vi "Finish.vi"   [LabVIEW 2017]
doc: "This VI is called just before exiting. It is expected to close I/O refnum, save collected data, etc."
uses:
  <vilib>/Rock Robotics/WPI/Utilities/WPI_GetSetVariantRefNum.vi
types:
  T1 = typedef "WPI_MotorControlDeviceRef.ctl" = cluster{"DeviceStatus":errorcluster, "Type":T2, "PWM":cluster{"PWM Channel":T3, "DeadBand":T4}, "CAN":cluster{"Device Number":u8, "SetOutput VI Ref":variant, "GetOutput VI Ref":variant, "Enable VI Ref":variant, "Disable VI Ref":variant, "Data":variant}, "Invert":bool, "DIO PWM":cluster{"PWM \"Enable\" Channel":T3, "DIOChannel":T5, "PWM Rate":dbl}}
  T2 = typedef "WPI_MotorControlType.ctl" = enum16{"PWM", "CAN", "DIO PWM"}
  T3 = typedef "FPGA_DIOPWMChannel.ctl" = enum8{"PWM 0", "PWM 1", "PWM 2", "PWM 3", "PWM 4", "PWM 5", "PWM 6", "PWM 7", "PWM 8", "PWM 9", "PWM MXP 0", "PWM MXP 1", "PWM MXP 2", "PWM MXP 3", "PWM MXP 4", "PWM MXP 5", "PWM MXP 6", "PWM MXP 7", "PWM MXP 8", "PWM MXP 9", "Invalid"}
  T4 = typedef "WPI_PWMDeadband.ctl" = cluster{"Name":string, "maxPositivePwm":i32, "minPositivePwm":i32, "centerPwm":i32, "maxNegativePwm":i32, "minNegativePwm":i32, "angularRange":u16}
  T5 = typedef "FPGA_DIOChannel.ctl" = enum8{"DIO 0", "DIO 1", "DIO 2", "DIO 3", "DIO 4", "DIO 5", "DIO 6", "DIO 7", "DIO 8", "DIO 9", "DIO MXP 0", "DIO MXP 1", "DIO MXP 2", "DIO MXP 3", "DIO MXP 4", "DIO MXP 5", "DIO MXP 6", "DIO MXP 7", "DIO MXP 8", "DIO MXP 9", "DIO MXP 10", "DIO MXP 11", "DIO MXP 12", "DIO MXP 13", "DIO MXP 14", "DIO MXP 15", "SPI Port CS1", "SPI Port CS2", "SPI Port CS3", "SPI Port MISO", "SPI Port MOSI", "Invalid"}
  T6 = typedef "WPI_SwitchDevRef.ctl" = cluster{"DevStatus":errorcluster, "DIO Channel":T5, "CntIndex":T7, "Normally Closed":bool}
  T7 = typedef "FPGA_CounterCtrSystemIndex.ctl" = enum8{"Ctr 0", "Ctr 1", "Ctr 2", "Ctr 3", "Ctr 4", "Ctr 5", "Ctr 6", "Ctr 7", "Invalid"}
  T8 = typedef "WPI_JoystickDevRef.ctl" = cluster{"Device":T9}
  T9 = typedef "WPI_JoystickDeviceEnum.ctl" = enum16{"USB 0", "USB 1", "USB 2", "USB 3", "USB 4", "USB 5"}
  T10 = typedef "WPI_RobotDriveDevRef.ctl" = cluster{"DevStatus":errorcluster, "Motors[]":T1[], "Square Inputs":bool, "Max Output":dbl}
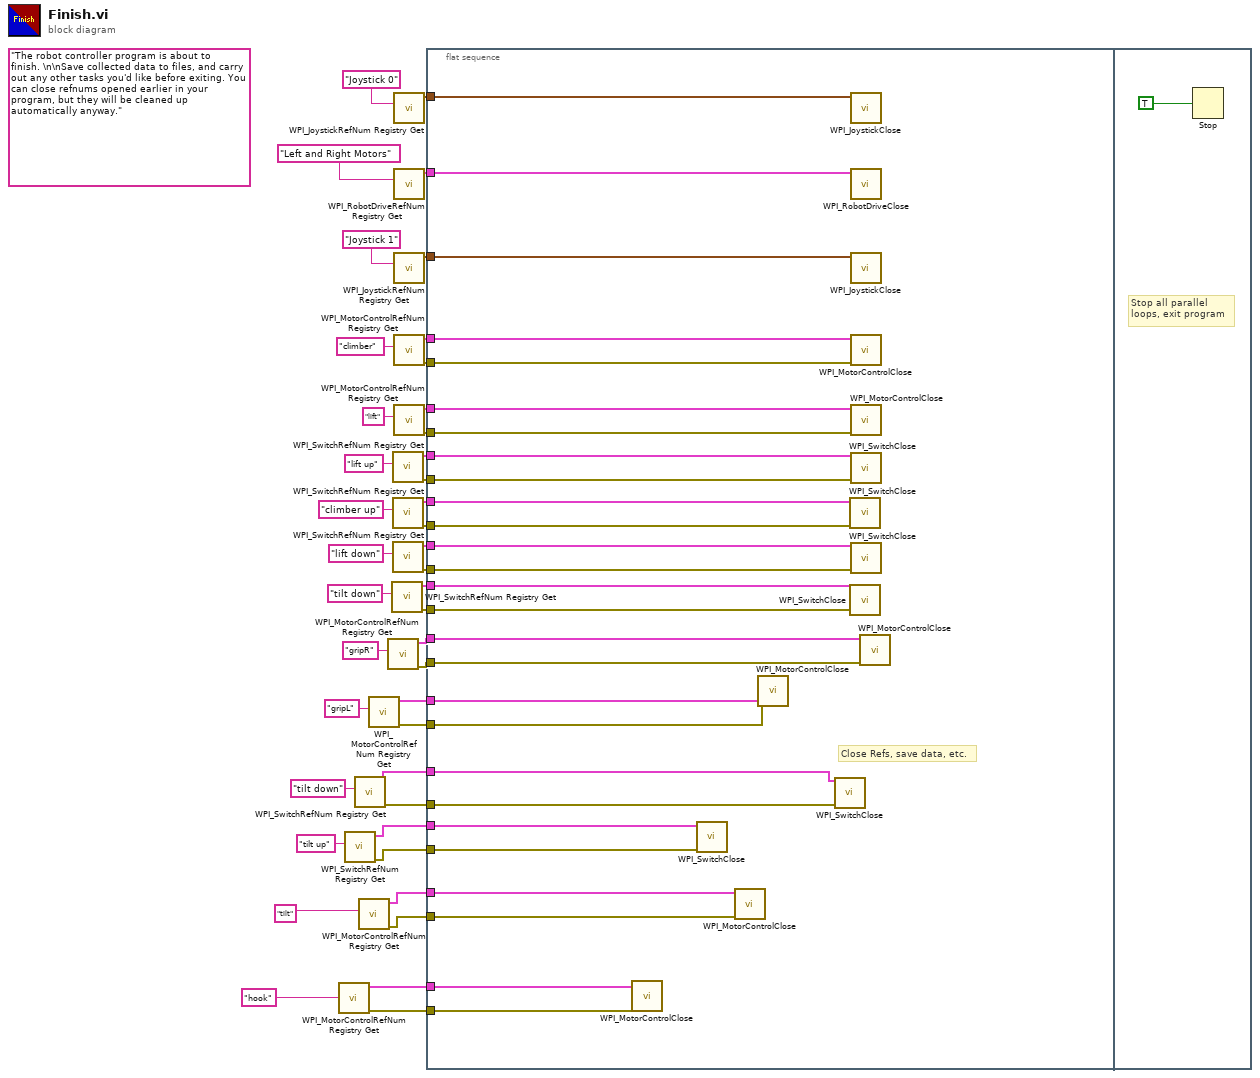
[diagram p0: block diagram]
diagram:
  (unwired) "The robot controller program is about to finish. \n\nSave collected data to files, and carry out any other tasks you'd like before exiting. You can close refnums opened earlier in your program, but they will be cleaned up automatically anyway."
  n1 = call <vilib>:"WPI_MotorControlRefNum Registry Get.vi"("refnum name"="hook") -> ("error out"=w1:errorcluster, "MotorControlDevRef"=w2:T1)  [unwired: 9 in]
  n2 = call <vilib>:"WPI_SwitchRefNum Registry Get.vi"("refnum name"="tilt up") -> ("error out"=w7:errorcluster, "SwitchDevRef"=w8:T6)  [unwired: 9 in]
  n3 = call <vilib>:"WPI_SwitchRefNum Registry Get.vi"("refnum name"="tilt down") -> ("error out"=w10:errorcluster, "SwitchDevRef"=w11:T6)  [unwired: 9 in]
  n4 = call <vilib>:"WPI_MotorControlRefNum Registry Get.vi"("refnum name"="tilt") -> ("error out"=w4:errorcluster, "MotorControlDevRef"=w5:T1)  [unwired: 9 in]
  n5 = call <vilib>:"WPI_MotorControlRefNum Registry Get.vi"("refnum name"="gripL") -> ("error out"=w13:errorcluster, "MotorControlDevRef"=w14:T1)  [unwired: 9 in]
  n6 = call <vilib>:"WPI_MotorControlRefNum Registry Get.vi"("refnum name"="gripR") -> ("error out"=w16:errorcluster, "MotorControlDevRef"=w17:T1)  [unwired: 9 in]
  n7 = call <vilib>:"WPI_SwitchRefNum Registry Get.vi"("refnum name"="tilt down") -> ("error out"=w23:errorcluster, "SwitchDevRef"=w25:T6)  [unwired: 9 in]
  n8 = call <vilib>:"WPI_SwitchRefNum Registry Get.vi"("refnum name"="lift up") -> ("error out"=w29:errorcluster, "SwitchDevRef"=w30:T6)  [unwired: 9 in]
  n9 = call <vilib>:"WPI_SwitchRefNum Registry Get.vi"("refnum name"="climber up") -> ("error out"=w27:errorcluster, "SwitchDevRef"=w28:T6)  [unwired: 9 in]
  n10 = call <vilib>:"WPI_SwitchRefNum Registry Get.vi"("refnum name"="lift down") -> ("error out"=w24:errorcluster, "SwitchDevRef"=w26:T6)  [unwired: 9 in]
  n11 = call <vilib>:"WPI_JoystickRefNum Registry Get.vi"("refnum name"="Joystick 0") -> ("JoystickDevRef"=w39:T8)  [unwired: 1 in, 9 out]
  n12 = call <vilib>:"WPI_RobotDriveRefNum Registry Get.vi"("refnum name"="Left and Right Motors") -> ("RobotDriveDevRef"=w40:T10)  [unwired: 1 in, 9 out]
  n13 = call <vilib>:"WPI_JoystickRefNum Registry Get.vi"("refnum name"="Joystick 1") -> ("JoystickDevRef"=w37:T8)  [unwired: 1 in, 9 out]
  n14 = call <vilib>:"WPI_MotorControlRefNum Registry Get.vi"("refnum name"="climber") -> ("error out"=w35:errorcluster, "MotorControlDevRef"=w36:T1)  [unwired: 9 in]
  n15 = call <vilib>:"WPI_MotorControlRefNum Registry Get.vi"("refnum name"="lift") -> ("error out"=w33:errorcluster, "MotorControlDevRef"=w34:T1)  [unwired: 9 in]
  n16 = flat-sequence {
    tunnel: w40 -> [w69]
    tunnel: w39 -> [w68]
    tunnel: w37 -> [w67]
    tunnel: w36 -> [w66]
    tunnel: w35 -> [w65]
    tunnel: w34 -> [w64]
    tunnel: w33 -> [w63]
    tunnel: w30 -> [w62]
    tunnel: w29 -> [w61]
    tunnel: w28 -> [w60]
    tunnel: w27 -> [w59]
    tunnel: w26 -> [w58]
    tunnel: w25 -> [w57]
    tunnel: w24 -> [w56]
    tunnel: w23 -> [w55]
    tunnel: w17 -> [w54]
    tunnel: w16 -> [w53]
    tunnel: w14 -> [w52]
    tunnel: w13 -> [w51]
    tunnel: w11 -> [w50]
    tunnel: w10 -> [w49]
    tunnel: w8 -> [w48]
    tunnel: w7 -> [w47]
    tunnel: w5 -> [w46]
    tunnel: w4 -> [w45]
    tunnel: w2 -> [w44]
    tunnel: w1 -> [w43]
    frame #0 {
      # "Close Refs, save data, etc."
      n17 = call <vilib>:"WPI_MotorControlClose.vi"("error in"=w43, "MotorControlDevRef"=w44) -> ()  [unwired: 9 in, 1 out]
      n18 = call <vilib>:"WPI_SwitchClose.vi"("error in (no error)"=w47, "SwitchDevRef"=w48) -> ()  [unwired: 9 in, 1 out]
      n19 = call <vilib>:"WPI_MotorControlClose.vi"("error in"=w45, "MotorControlDevRef"=w46) -> ()  [unwired: 9 in, 1 out]
      n20 = call <vilib>:"WPI_MotorControlClose.vi"("error in"=w51, "MotorControlDevRef"=w52) -> ()  [unwired: 9 in, 1 out]
      n21 = call <vilib>:"WPI_SwitchClose.vi"("error in (no error)"=w49, "SwitchDevRef"=w50) -> ()  [unwired: 9 in, 1 out]
      n22 = call <vilib>:"WPI_SwitchClose.vi"("error in (no error)"=w59, "SwitchDevRef"=w60) -> ()  [unwired: 9 in, 1 out]
      n23 = call <vilib>:"WPI_SwitchClose.vi"("error in (no error)"=w55, "SwitchDevRef"=w57) -> ()  [unwired: 9 in, 1 out]
      n24 = call <vilib>:"WPI_JoystickClose.vi"("JoystickDevRef"=w68) -> ()  [unwired: 11 out]
      n25 = call <vilib>:"WPI_RobotDriveClose.vi"("RobotDriveDevRef"=w69) -> ()  [unwired: 1 in, 10 out]
      n26 = call <vilib>:"WPI_JoystickClose.vi"("JoystickDevRef"=w67) -> ()  [unwired: 11 out]
      n27 = call <vilib>:"WPI_MotorControlClose.vi"("error in"=w65, "MotorControlDevRef"=w66) -> ()  [unwired: 9 in, 1 out]
      n28 = call <vilib>:"WPI_MotorControlClose.vi"("error in"=w63, "MotorControlDevRef"=w64) -> ()  [unwired: 9 in, 1 out]
      n29 = call <vilib>:"WPI_SwitchClose.vi"("error in (no error)"=w61, "SwitchDevRef"=w62) -> ()  [unwired: 9 in, 1 out]
      n30 = call <vilib>:"WPI_SwitchClose.vi"("error in (no error)"=w56, "SwitchDevRef"=w58) -> ()  [unwired: 9 in, 1 out]
      n31 = call <vilib>:"WPI_MotorControlClose.vi"("error in"=w53, "MotorControlDevRef"=w54) -> ()  [unwired: 9 in, 1 out]
    }
    frame #1 {
      # "Stop all parallel\nloops, exit program"
      n32 = Stop(stop? (T)=TRUE ("Quit")) -> ()
    }
  }
